vi "EEG Features Extraction.vi"() -> ()   [LabVIEW 2016]
uses:
  _vlib/EF_FrequencyFilter.ctl
  _vlib/EF_SpatialFilter.ctl
  _vlib/EF_FeatureExtractionMethods.ctl
  _XML_EEG_Features/XML_FF_Trial.ctl
  _XML_EEG_File_Parser/_vlib/XML_EEG_File.lvclass
  _XML_EEG_Features/XML_FF_Header.ctl
  <vilib>/xml/Load XML File.vi
  <vilib>/xml/Close Reference(Node).vi
  <vilib>/xml/NI_XML.lvlib
  _XML_EEG_Features/XML_EEG_Features.lvlib
  Feature Extraction.lvlib
panel:
  in  "Tab Control":enum32{"Настройка", "Обработка"}(tab)
  in  "Tab Control 2":T1(tab)=enum."Формирование признаков"
  in  "EOG channels":i32[](array[numeric])=[22, 23, 24] caption="Каналы с электроокулограммой (ЭОГ)" min=0 max=256 step=1
  in  "CSP params":path caption="Путь к файлу с параметрами CSP-фильтра"
  in  "SpatialFilter":T2=enum."Common Average Reference" caption="Метод пространственной фильтрации"
  in  "low cutoff freq":dbl=0.5 caption="Нижняя граница полосы пропускания, Гц"
  in  "high cutoff freq":dbl=50.0 caption="Верхняя граница полосы пропускания, Гц"
  in  "FrequencyFilter":T3 caption="Метод частотной фильтрации"
  in  "Parameter #2":dbl=30.0 caption="Параметр #2" min=-1000.0 max=1000.0 step=0.1
  in  "Parameter #1":dbl caption="Параметр #1" min=-1000.0 max=1000.0 step=0.1
  in  "FeatureExtractionMethod":T4=enum."EEG Bicoherence" caption="Метод формирования признаков"
  in  "Start":bool
  out "Features":dbl[][](array[numeric])=[[91.6357924667573], [76.75495965471536], [95.03921243134478], [112.48185823441702], [111.83881597008215], [103.0579992170672], [51.68063842706969], [71.73918271243171], [91.4461695420327], [114.20714437739215], [106.11029840698885], [94.05121079387746], [67.64386344076077], [71.25840412068811], [84.41739823475822], [97.28988156008135], [89.52024761342335], [84.18174370644296], [75.7593978088008], [78.79611354745819], [71.17687035099024], [66.48806089004955]] caption="Характерные признаки сигнала"
  out "dataset label":string="Tongue - cue onset (BCI experiment)" caption="Метка класса"
  out "current dataset":i32=12 caption="Проба"
  out "sampling rate":dbl=250.0 caption="Частота дискретизации"
  out "number of datasets":i32=12 caption="Число проб в файле"
  out "Processing File":path=path "E:/BCI_Project/_EEG_Data/A01/train/Tongue - cue onset (BCI experiment)-5.xml" caption="Обрабатываемый файл"
  out "feature vector length":i32=22 caption="Длина вектора признаков"
  # "This VI is a part of BCI Design library, http://www.ru-bci.org \nCopyright © 2020, Sotnikov Peter, All rights reserved. License: GNU GPLv3"
  # "(с) Sotnikov P, 2016"
  # "Параметры метода"
  # "Параметры метода"
  # "Параметры метода"
  # "Метод Amplitude Entropy:\nПараметр #1 - Минимальное возможное значение амплитуды сигнала, мкВ\nПараметр #2 - Максимальное возможное значение амплитуды сигнала, мкВ\nМетоды EEG Spectrum, Wavelet Scalogram, EEG Bicoherence:\nПараметр #1 - Нижняя граница частотного диапазона, Гц\nПараметр #2 - Верхняя граница частотного диапазона, Гц\nМетод Signal Downsampling:\nПараметр #1 - Коэффициент понижения частоты выборок\nМетод Vector Autoregressive Model:\nПараметр #1 - Порядок модели авторегрессии"
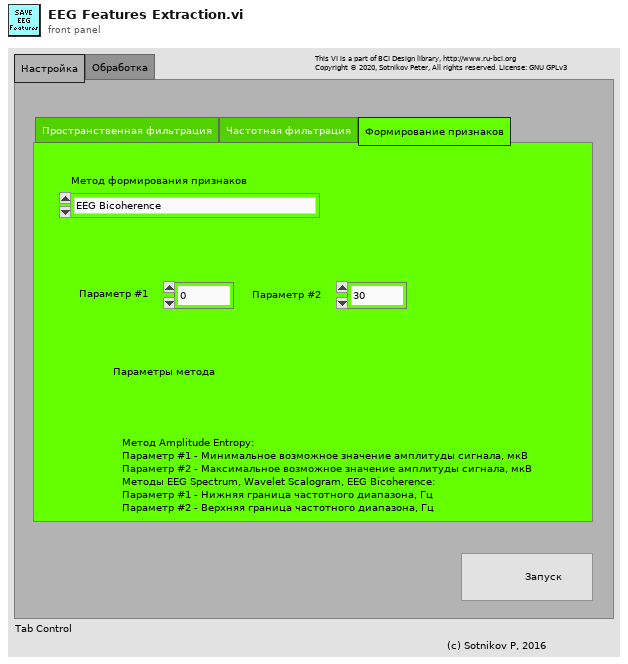
[diagram p1: front panel]
types:
  T1 = enum32{"Пространственная фильтрация", "Частотная фильтрация", "Формирование признаков"}
  T2 = typedef "Feature Extraction.lvlib/EF_SpatialFilter.ctl" = enum16{"No Filter", "Common Average Reference", "Common Spatial Pattern Filter", "Removal of EOG Artifacts"}
  T3 = typedef "Feature Extraction.lvlib/EF_FrequencyFilter.ctl" = enum16{"No Filter", "Kaiser Filter"}
  T4 = typedef "Feature Extraction.lvlib/EF_FeatureExtractionMethods.ctl" = enum16{"Amplitude Variance", "Amplitude Entropy", "EEG Spectrum (FourierTransform)", "EEG Spectrum (WaveletTransform)", "Spectral Power of EEG Rhythms (FourierTransform)", "Spectral Power of EEG Rhythms (WaveletTransform)", "Wavelet Scalogram", "Signal Downsampling", "Vector Autoregressive Model", "EEG Bicoherence"}
  T5 = typedef "XML_EEG_Features.lvlib/XML_FF_Trial.ctl" = cluster{"ClassLabel":string, "FeatureVector":dbl[]}
  T6 = typedef "XML_EEG_Features.lvlib/XML_FF_Header.ctl" = cluster{"NumberOfTrials":i32, "NumberOfClasses":i32, "FeatureVectorLength":i32, "FeatureExtractionMethod":string}
  T7 = cluster{"SpatialFilter":T2, "CSP params":path, "FrequencyFilter":T3, "low cutoff freq":dbl, "high cutoff freq":dbl}
  T8 = cluster{"FeatureExtractionMethod":T4, "Parameter #1":dbl, "Parameter #2":dbl}
  T9 = typedef "XML_EEG_File_Parser.lvlib/XML_EEG_Header.ctl" = cluster{"Attributes":cluster{"ChannelDataType":string, "NumberOfChannels":i32, "SampleRateHz":dbl, "MarkerChannel":i32}, "Body":cluster{"PatientSpecificData":string, "NumberOfDatasets":i32, "Channels":string[]}}
  T10 = typedef "XML_EEG_File_Parser.lvlib/XML_EEG_Dataset.ctl" = cluster{"Attributes":cluster{"NumberOfSamples":i32, "StartDateTime":timestamp}, "Body":cluster{"MarkerValue":string, "Channels":waveform(dbl)[]}}
  T11 = typedef "EF_FeatureExtractionMethods.ctl" = enum16{"Amplitude Variance", "Amplitude Entropy", "EEG Spectrum (FourierTransform)", "EEG Spectrum (WaveletTransform)", "Spectral Power of EEG Rhythms (FourierTransform)", "Spectral Power of EEG Rhythms (WaveletTransform)", "Wavelet Scalogram", "Signal Downsampling", "Vector Autoregressive Model", "EEG Bicoherence"}
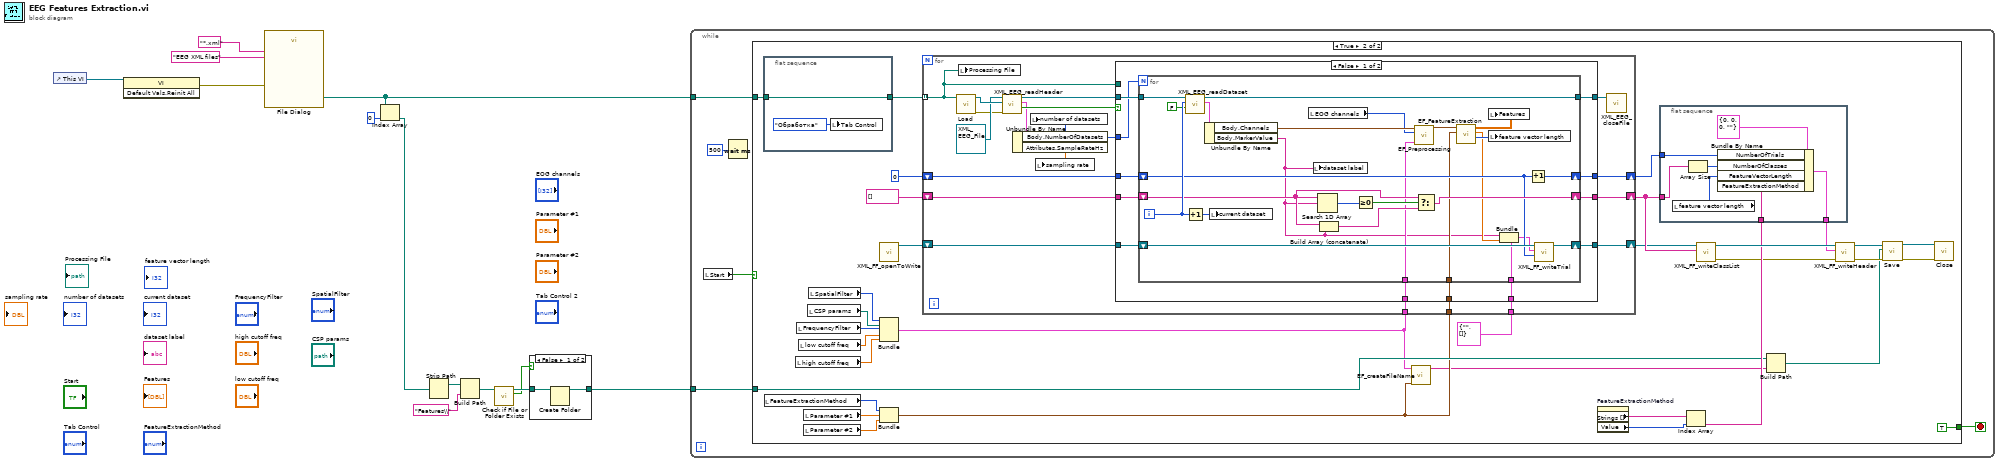
[diagram p0: block diagram]
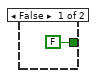
[diagram p2: hidden frame]
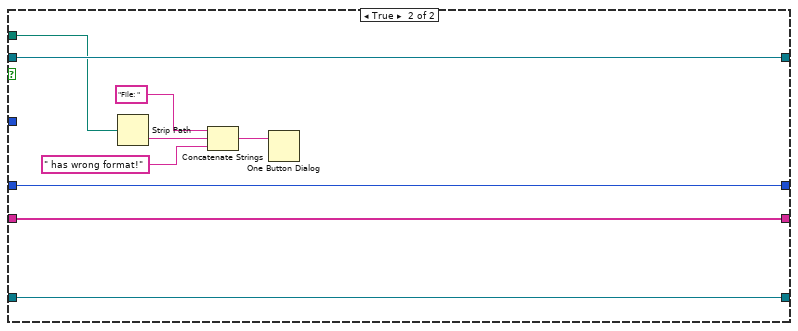
[diagram p3: hidden frame]
diagram:
  n1 = control-ref of="This VI"() -> (w12:refnum<vi>)
  n2 = invoke class="VI" method="Default Vals.Reinit All"(reference=w12) -> (error out=w2:errorcluster)  [unwired: 2 in, 2 out]
  n3 = call "File Dialog"("error in"=w2, "pattern (all files)"="*.xml", "pattern label"="EEG XML files") -> ("selected paths"=w4:path[])  [unwired: 9 in, 3 out]
  n4 = Index Array(array=w4, index=0) -> (element=w1:path)
  n5 = Strip Path(path=w1) -> (stripped path=w9:path)  [unwired: 1 out]
  n6 = Build Path(base path=w9, name or relative path="Features\\") -> (appended path=w7:path)
  n7 = call <vilib>:"Check if File or Folder Exists.vi"("path"=w7) -> ("file or folder exists?"=w5:bool, "dup path"=w6:path)  [unwired: 8 in, 1 out]
  n8 = case shown="False" w5 {
    tunnel: w6 -> [w15 w16]
    tunnel: [w14 w16] -> w3
    frame False {
      n9 = Create Folder(path (use dialog)=w15) -> (created path=w14:path)  [unwired: 2 in, 2 out]
    }
    frame True {
    }
  }
  n10 = while {
    tunnel: w4 -> [w20]
    tunnel: w3 -> [w19]
    stop <- w17 stop-if-true
    n11 = local read "Start"() -> (w21:bool)
    n12 = Wait (ms)(milliseconds to wait=u32 500) -> ()  [unwired: 1 out]
    n13 = case shown="True" w21 {
      tunnel: w20 -> [_ w34]
      tunnel: w19 -> [_ w28]
      tunnel: [FALSE TRUE] -> w17
      frame False {
      }
      frame True {
        n14 = flat-sequence {
          tunnel: w34 -> [w64]
          tunnel: [w64] -> w33
          frame #0 {
            n15 = local write "Tab Control"(enum32{"Настройка", "Обработка"}."Обработка" ("Tab Control")) -> ()
          }
        }
        n16 = local read "FeatureExtractionMethod"() -> (w32:T4)
        n17 = local read "high cutoff freq"() -> (w50:dbl)
        n18 = local read "FrequencyFilter"() -> (w52:T3)
        n19 = local read "low cutoff freq"() -> (w51:dbl)
        n20 = local read "Parameter #1"() -> (w31:dbl)
        n21 = local read "Parameter #2"() -> (w23:dbl)
        n22 = local read "CSP params"() -> (w53:path)
        n23 = local read "SpatialFilter"() -> (w54:T2)
        n24 = call "XML_FF_openToWrite.vi"() -> ("DOM document out"=w38:refnum<k20>)  [unwired: 10 in, 1 out]
        n25 = Bundle("SpatialFilter"=w54, "CSP params"=w53, "FrequencyFilter"=w52, "low cutoff freq"=w51, "high cutoff freq"=w50) -> (w26:T7)  [unwired: 1 in]
        n26 = Bundle("FeatureExtractionMethod"=w32, "Parameter #1"=w31, "Parameter #2"=w23) -> (w25:T8)  [unwired: 1 in]
        n27 = for {
          tunnel: w33 -> [w75] mode=indexing
          shift-right: [w73] -> w44
          shift-left: string[] [] -> [w74]
          tunnel: w26 -> [w72]
          shift-right: [w71] -> w37
          shift-left: w38 -> [w70]
          shift-right: [w68] -> w35
          shift-left: 0 -> [w69]
          tunnel: w25 -> [w66]
          tunnel: T5 {"ClassLabel"="", "FeatureVector"=[]} ("XML_FF_Trial") -> [w65]
          n28 = call-poly <vilib>:"Load.vi"("path to XML document"=w75) -> ("DOM document out"=w83:refnum<k20>, "error out"=w81:errorcluster)  [unwired: 12 in, 1 out]
          n29 = local write "Processing File"(w75) -> ()
          n30 = call "XML_EEG_readHeader.vi"("error in (no error)"=w81, "DOM document in"=w83, "XML_EEG_Class in"=refnum<class "XML_EEG_File.lvclass"> refnum ("XML_EEG_File_Parser.lvlib:XML_EEG_File.lvclass")) -> ("Errors?"=w80:bool, "XML Header out"=w78:T9, "XML_EEG_Class out"=w79:refnum<class "XML_EEG_File.lvclass">)  [unwired: 6 in]
          n31 = Unbundle By Name(w78) -> ("Body.NumberOfDatasets"=w67:i32, "Attributes.SampleRateHz"=w77:dbl)
          n32 = local write "number of datasets"(w67) -> ()
          n33 = local write "sampling rate"(w77) -> ()
          n34 = case shown="False" w80 {
            tunnel: w79 -> [w95 w130]
            tunnel: w67 -> [w94 _]
            tunnel: [w93 w130] -> w76
            tunnel: w75 -> [_ w129]
            tunnel: w74 -> [w92 w124]
            tunnel: [w91 w124] -> w73
            tunnel: w72 -> [w90 _]
            tunnel: w70 -> [w89 w123]
            tunnel: [w88 w123] -> w71
            tunnel: w69 -> [w87 w122]
            tunnel: [w86 w122] -> w68
            tunnel: w66 -> [w85 _]
            tunnel: w65 -> [w84 _]
            frame False {
              n35 = for {
                N: w94 -> [_]
                tunnel: w95 -> [w121]
                tunnel: [w116] -> w93
                shift-right: [w111] -> w91
                shift-left: w92 -> [w113]
                tunnel: w90 -> [w106]
                shift-right: [w109] -> w88
                shift-left: w89 -> [w110]
                shift-right: [w108] -> w86
                shift-left: w87 -> [w107]
                tunnel: w85 -> [w104]
                tunnel: w84 -> [w99]
                i -> [w120]
                n36 = call "XML_EEG_readDataset.vi"("Add offset?"=FALSE, "DatasetNumber"=w120, "XML_EEG_File in"=w121) -> ("XML Dataset out"=w117:T10, "XML_EEG_File out"=w116:refnum<class "XML_EEG_File.lvclass">)  [unwired: 6 in, 1 out]
                n37 = Increment(x=w120) -> (x+1=w119:i32)
                n38 = Unbundle By Name(w117) -> ("Body.Channels"=w97:waveform(dbl)[], "Body.MarkerValue"=w98:string)
                n39 = local write "current dataset"(w119) -> ()
                n40 = local read "EOG channels"() -> (w96:i32[])
                n41 = local write "dataset label"(w98) -> ()
                n42 = Search 1D Array(1D array=w113, element=w98) -> (index of element=w115:i32)  [unwired: 1 in]
                n43 = Build Array (concatenate)(w113, w98) -> (w112:string[])
                n44 = Greater Or Equal To 0?(x=w115) -> (x >= 0?=w114:bool)
                n45 = call "EF_Preprocessing.vi"("Preprocessing params"=w106, "EOG channels"=w96, "EEG data in"=w97) -> ("EEG data out"=w105:waveform(dbl)[])  [unwired: 8 in]
                n46 = Select(t=w113, s=w114, f=w112) -> (s? t:f=w111:string[])
                n47 = call "EF_FeatureExtraction.vi"("FeatureExtractionParams"=w104, "Array Of Waveforms in"=w105) -> ("FeatureVector Length"=w102:i32, "FeatureVector"=w101:dbl[], "Feature Matrix"=w103:dbl[][])  [unwired: 6 in, 1 out]
                n48 = local write "Features"(w103) -> ()
                n49 = local write "feature vector length"(w102) -> ()
                n50 = Bundle(cluster=w99, "ClassLabel"=w98, "FeatureVector"=w101) -> (w100:T5)
                n51 = Increment(x=w107) -> (x+1=w108:i32)
                n52 = call "XML_FF_writeTrial.vi"("Trial Number"=w107, "XML_FF_Trial"=w100, "DOM document in"=w110) -> ("DOM document out"=w109:refnum<k20>)  [unwired: 7 in, 1 out]
              }
            }
            frame True {
              n53 = Strip Path(path=w129) -> (name=w128:string)  [unwired: 1 out]
              n54 = Concatenate Strings("File: " ("string"), w128, " has wrong format!" ("string")) -> (w125:string)
              n55 = One Button Dialog(message=w125) -> ()  [unwired: 1 in, 1 out]
            }
          }
          n56 = call "XML_EEG_closeFile.vi"("XML_EEG_File.lvclass"=w76) -> ()  [unwired: 10 in, 1 out]
        }
        n57 = call "EF_createFileName.vi"("FeatureExtractionParams"=w25, "Preprocessing params"=w26) -> ("FeaturesFile Name"=w24:string)  [unwired: 9 in]
        n58 = property on="FeatureExtractionMethod" class="Enum (strict)"() -> ("Strings []"=w43:string[], "Value"=w42:T11)  [unwired: 2 in, 2 out]
        n59 = flat-sequence {
          tunnel: w44 -> [w56]
          tunnel: w41 -> [w60]
          tunnel: [w59] -> w39
          tunnel: w35 -> [w58]
          frame #0 {
            n60 = local read "feature vector length"() -> (w57:i32)
            n61 = Array Size(array=w56) -> (size(s)=w61:i32)
            n62 = Bundle By Name(cluster=T6 {"NumberOfTrials"=0, "NumberOfClasses"=0, "FeatureVectorLength"=0, "FeatureExtractionMethod"=""} ("XML_FF_Header"), "NumberOfTrials"=w58, "NumberOfClasses"=w61, "FeatureVectorLength"=w57, "FeatureExtractionMethod"=w60) -> (w59:T6)
          }
        }
        n63 = Index Array(array=w43, index=w42) -> (element=w41:string)
        n64 = call "XML_FF_writeClassList.vi"("ClassList"=w44, "DOM document in"=w37) -> ("error out"=w40:errorcluster, "DOM document out"=w49:refnum<k20>)  [unwired: 8 in]
        n65 = Build Path(base path=w28, name or relative path=w24) -> (appended path=w27:path)
        n66 = call "XML_FF_writeHeader.vi"("error in (no error)"=w40, "XML_FF_Header"=w39, "DOM document in"=w49) -> ("error out"=w47:errorcluster, "DOM document out"=w48:refnum<k20>)  [unwired: 7 in]
        n67 = call <vilib>:"Save.vi"("error in (no error)"=w47, "XML file path"=w27, "DOM document in"=w48) -> ("error out"=w45:errorcluster, "DOM document out"=w46:refnum<k20>)  [unwired: 6 in, 1 out]
        n68 = call-poly <vilib>:"Close.vi"("error in (no error)"=w45, "node"=w46) -> ()  [unwired: 7 in, 1 out]
      }
    }
  }
